vi "MyRIO_Queue.vi"() -> (0 "error out":errorcluster, 3 "Queues out":T1, 5 "Error Conneciton":bool)   [LabVIEW 2019]
uses:
  TypeDef/#TypeDef_MyRIO_Queues.ctl
  Data Processing/TypeDef/#TypeDef_PropFromDAtoDP.ctl
  Communication/TypeDef/#TypeDef_FromPCtoMR.ctl
  Communication/TypeDef/#TypeDef_Command.ctl
  Communication/TypeDef/#TypeDef_ErrorHandler_prop.ctl
  Communication/TypeDef/#TypeDef_FromMRtoPC.ctl
  Communication/TypeDef/#TypeDef_PropGraph.ctl
  Communication/TypeDef/#TypeDef_PropertiesToSave.ctl
  Communication/TypeDef/#TypeDef_EnumConnection.ctl
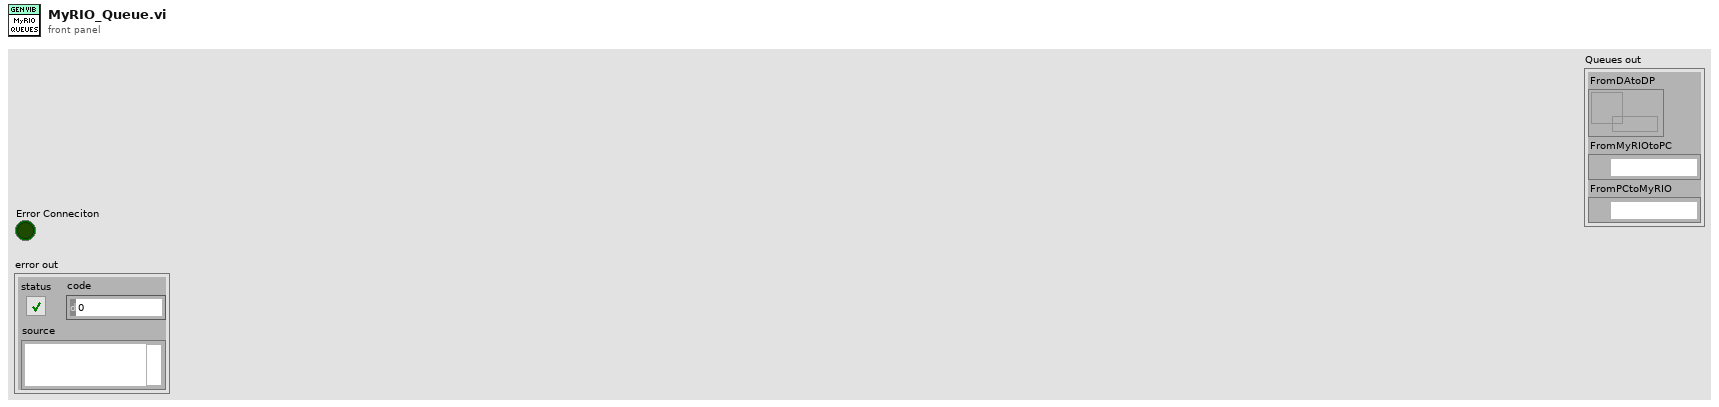
[diagram p1: front panel]
types:
  T1 = typedef "#TypeDef_MyRIO_Queues.ctl" = cluster{"FromDAtoDP":refnum<queue>, "FromMyRIOtoPC":refnum<k21>, "FromPCtoMyRIO":refnum<k21>}
  T2 = typedef "#TypeDef_EnumConnection.ctl" = enum16{"Try to Connect PCMyRio", "Try to Connect MyRioPC", "Send queues", "Error"}
  T3 = typedef "#TypeDef_FromPCtoMR.ctl" = cluster{"Command":T4, "Error?":bool, "Stop":bool, "StopPomiar":bool, "Name":string, "FilesPath":path, "ErrorHandler":T5, "Fs":dbl}
  T4 = typedef "#TypeDef_Command.ctl" = enum16{"Start", "End"}
  T5 = typedef "#TypeDef_ErrorHandler_prop.ctl" = cluster{"Threads":enum16{"Acquisistion", "Data Operation", "Save File"}, "ClearError":bool, "Error Out ":errorcluster, "Error":bool}
  T6 = typedef "#TypeDef_FromMRtoPC.ctl" = cluster{"Accessibility":T3, "PropGraph":T7, "No Data?":bool, "WaveformData":waveform(dbl)[]}
  T7 = typedef "#TypeDef_PropGraph.ctl" = cluster{"Raw Data":dbl[][], "Poperties":T8, "Power Spectrum / PSD":cluster{"f0":dbl, "df":dbl, "magnitude":dbl[]}[]}
  T8 = typedef "#TypeDef_PropertiesToSave.ctl" = cluster{"RMS values":dbl[], "Max":dbl[], "Min":dbl[], "A(8)":dbl[], "t":dbl, "A(8) Axis":dbl, "Aw":dbl[], "Ak 30min":dbl, "Ak_axis":i32, "Spec":cluster{"f0":dbl, "df":dbl, "magnitude":dbl[]}[]}
  T9 = typedef "#TypeDef_PropFromDAtoDP.ctl" = cluster{"Accessibility":T3, "RawData":dbl[][], "Counter":i32, "Fs":dbl}
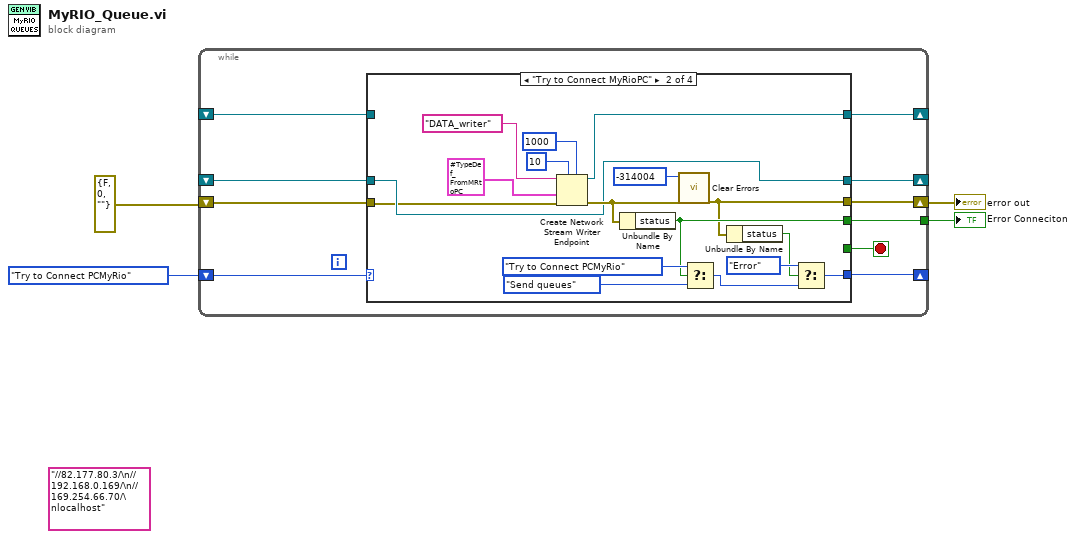
[diagram p0: block diagram]
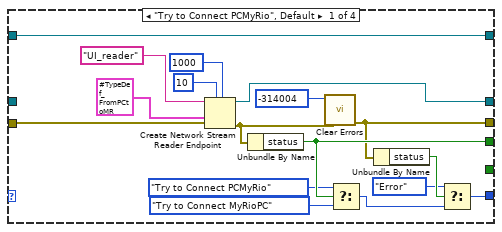
[diagram p2: hidden frame]
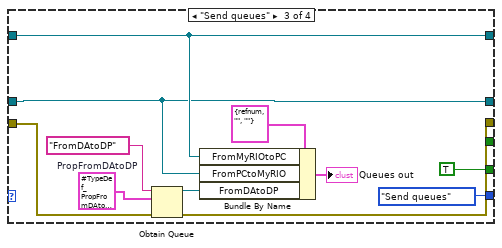
[diagram p3: hidden frame]
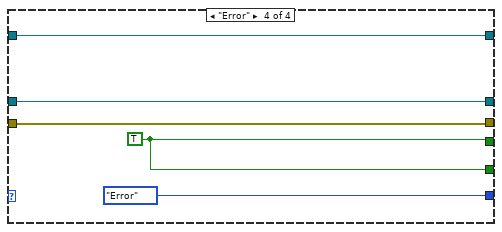
[diagram p4: hidden frame]
diagram:
  (unwired) "//82.177.80.3/\n//192.168.0.169/\n//169.254.66.70/\nlocalhost"
  n1 = while {
    shift-right: [w13] -> w3
    shift-left: errorcluster {"status"=FALSE, "code"=0, "source"=""} ("error out") -> [w12]
    shift-right: [w11] -> _
    shift-left: _ -> [w5]
    shift-right: [w10] -> _
    shift-left: _ -> [w9]
    shift-right: [w6] -> _
    shift-left: #TypeDef_EnumConnection."Try to Connect PCMyRio" -> [w14]
    tunnel: [w7] -> w2
    stop <- w8 stop-if-true
    n2 = case shown="\"Try to Connect MyRioPC\"" w14 {
      tunnel: [w20 w35 w53 w64] -> w13
      tunnel: w12 -> [w15 w33 w54 w64]
      tunnel: [w28 w45 w50 w62] -> w11
      tunnel: [w23 w46 w49 w61] -> w10
      tunnel: w5 -> [w28 _ w50 w62]
      tunnel: w9 -> [_ w46 w49 w61]
      tunnel: [_ _ TRUE w63] -> w8
      tunnel: [w27 w36 _ w63] -> w7
      tunnel: [w17 w37 #TypeDef_EnumConnection."Send queues" #TypeDef_EnumConnection."Error"] -> w6
      frame "Try to Connect PCMyRio", Default {
        n3 = Create Network Stream Reader Endpoint(5:1000 ("timeout in ms (-1)"), 7:10 ("writer buffer size"), 8:w15, 9:T3 {"Command"=enum."End", "Error?"=FALSE, "Stop"=FALSE, "StopPomiar"=FALSE, "Name"="", "FilesPath"=path "", "ErrorHandler"={"Threads"=enum."Acquisistion", "ClearError"=FALSE, "Error Out "={"status"=FALSE, "code"=0, "source"=""}, "Error"=FALSE}, "Fs"=0.0} ("PCtoMyRio"), 11:"UI_reader" ("writer name")) -> (0:w31:errorcluster, 3:w23:refnum<k21>)  [unwired: 2 in]
        n4 = Unbundle By Name(w31) -> ("status"=w27:bool)
        n5 = call <vilib>:"Clear Errors.vi"("error in (no error)"=w31, "specific error code to clear (0: all)"=-314004) -> ("error out"=w20:errorcluster)  [unwired: 4 in, 1 out]
        n6 = Select(t=#TypeDef_EnumConnection."Try to Connect PCMyRio", s=w27, f=#TypeDef_EnumConnection."Try to Connect MyRioPC") -> (s? t:f=w18:T2)
        n7 = Unbundle By Name(w20) -> ("status"=w19:bool)
        n8 = Select(t=#TypeDef_EnumConnection."Error", s=w19, f=w18) -> (s? t:f=w17:T2)
      }
      frame "Try to Connect MyRioPC" {
        n9 = Create Network Stream Writer Endpoint(5:1000 ("timeout in ms (-1)"), 7:10 ("writer buffer size"), 8:w33, 9:T6 {"Accessibility"={"Command"=enum."End", "Error?"=FALSE, "Stop"=FALSE, "StopPomiar"=FALSE, "Name"="", "FilesPath"=path "", "ErrorHandler"={"Threads"=enum."Acquisistion", "ClearError"=FALSE, "Error Out "={"status"=FALSE, "code"=0, "source"=""}, "Error"=FALSE}, "Fs"=0.0}, "PropGraph"={"Raw Data"=[[0.0], [0.0234375], [0.9609375]], "Poperties"={"RMS values"=[], "Max"=[], "Min"=[], "A(8)"=[], "t"=0.0, "A(8) Axis"=0.0, "Aw"=[], "Ak 30min"=0.0, "Ak_axis"=0, "Spec"=[]}, "Power Spectrum / PSD"=[]}, "No Data?"=FALSE, "WaveformData"=[]} ("FromMyRiOtoUI"), 11:"DATA_writer" ("writer name")) -> (0:w48:errorcluster, 3:w45:refnum<k21>)  [unwired: 2 in]
        n10 = Unbundle By Name(w48) -> ("status"=w36:bool)
        n11 = call <vilib>:"Clear Errors.vi"("error in (no error)"=w48, "specific error code to clear (0: all)"=-314004) -> ("error out"=w35:errorcluster)  [unwired: 4 in, 1 out]
        n12 = Select(t=#TypeDef_EnumConnection."Try to Connect PCMyRio", s=w36, f=#TypeDef_EnumConnection."Send queues") -> (s? t:f=w39:T2)
        n13 = Unbundle By Name(w35) -> ("status"=w34:bool)
        n14 = Select(t=#TypeDef_EnumConnection."Error", s=w34, f=w39) -> (s? t:f=w37:T2)
      }
      frame "Send queues" {
        w51 = T9 {"Accessibility"={"Command"=enum."End", "Error?"=FALSE, "Stop"=FALSE, "StopPomiar"=FALSE, "Name"="", "FilesPath"=path "", "ErrorHandler"={"Threads"=enum."Acquisistion", "ClearError"=FALSE, "Error Out "={"status"=FALSE, "code"=0, "source"=""}, "Error"=FALSE}, "Fs"=0.0}, "RawData"=[], "Counter"=0, "Fs"=0.0}  # PropFromDAtoDP
        n15 = Obtain Queue(name (unnamed)="FromDAtoDP", element data type=w51, error in (no error)=w54) -> (queue out=w52:refnum<queue>, error out=w53:errorcluster)  [unwired: 2 in, 1 out]
        n16 = Bundle By Name(cluster=T1 {"FromDAtoDP"=refnum, "FromMyRIOtoPC"="", "FromPCtoMyRIO"=""}, "FromMyRIOtoPC"=w50, "FromPCtoMyRIO"=w49, "FromDAtoDP"=w52) -> (→"Queues out":T1)
      }
      frame "Error" {
        w63 = TRUE
      }
    }
  }
  "error out" <- w3
  "Error Conneciton" <- w2
